vi "Compatibility Pulse Generation.vi"() -> ()   [LabVIEW 2023]
doc: "The Compatibility Pulse Generation example demonstrates how to generate a pulse on an external or RTSI trigger line. Use a pulse to control external events such as triggering a strobe light.\n\nThis example uses the IMAQdx driver to interface with a Camera Link frame grabber. It uses the NI-IMAQdx Compatibility for NI-IMAQ API to facilitate migration between the two drivers. The NI-IMAQdx VIs are drop-in replacements to existing NI-IMAQ VIs."
uses:
  <vilib>/vision/driver/NI_Vision_Acquisition_Software.lvlib
panel:
  in  "Camera Name":refnum<k21> caption="IMAQdx Session"
  in  "Trigger Type":u32(ring) items=["External"=0, "RTSI"=1, "ISO Out"=3]
  in  "Pulse Parameters":T1={"Pulse Delay"=0.1, "Pulse Width"=0.2, "Pulse Polarity"=enum."High True ", "Units"=enum."Seconds"} {"Pulse Width" format="%_6f"; "Pulse Delay" format="%_6f"}
  in  "Signal Type":u32(ring)=4 items=["External"=0, "RTSI "=1, "ISO In"=2, "Status"=4]
  in  "Signal Number":u32
  in  "Status Signal":u32(ring)=16 items=["Acquisition in progress"=15, "Acquisition done"=8, "Horizontal Synchronization Signal"=18, "Vertical Synchronization Signal"=19, "Frame start"=9, "Frame done"=10, "Immediate"=16]
  in  "Trigger Number":u32
  in  "Stop":bool
  out "Image":T2(plugin-control)
  # "Overview: Demonstrates how to generate a pulse or pulse train on one of the external or RTSI trigger lines of a Camera Link frame grabber board.\nRequirements: Vision Acquisition Software 18.0 or later, PCIe-1427, PCIe-1433, PXIe-1435, or PCIe-1437 frame grabber.\nInstructions: \n1. Select the Camera Name.\n2. Run the VI."
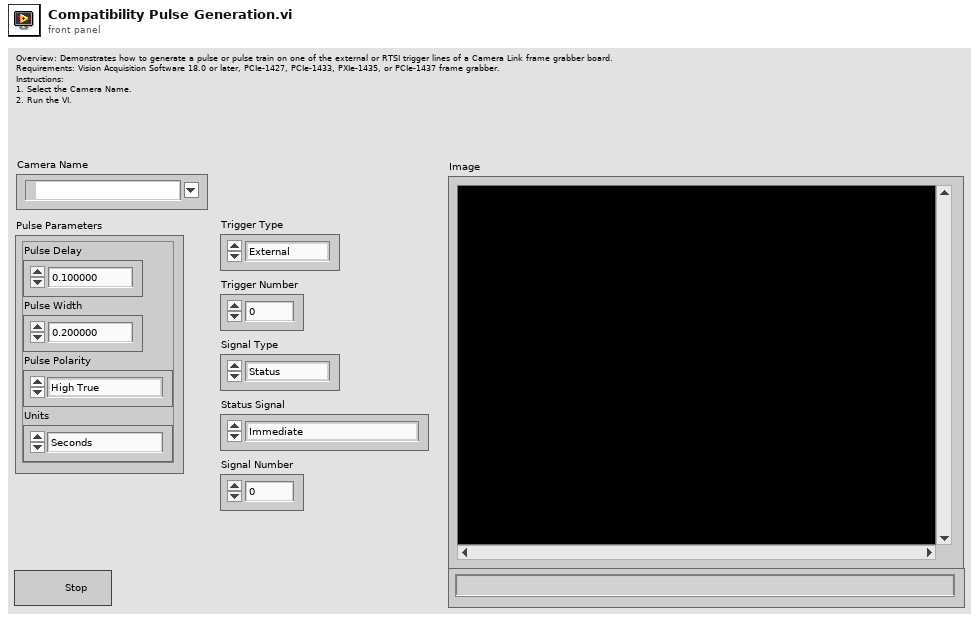
[diagram p1: front panel]
types:
  T1 = cluster{"Pulse Delay":dbl, "Pulse Width":dbl, "Pulse Polarity":enum16{"High True ", "Low True"}, "Units":enum16{"Seconds", "Scaled Encoder Counts"}}
  T2 = typedef "IMAQ Image.ctl" = refnum<image>
  T3 = typedef "IMAQdx.ctl" = refnum<k21>
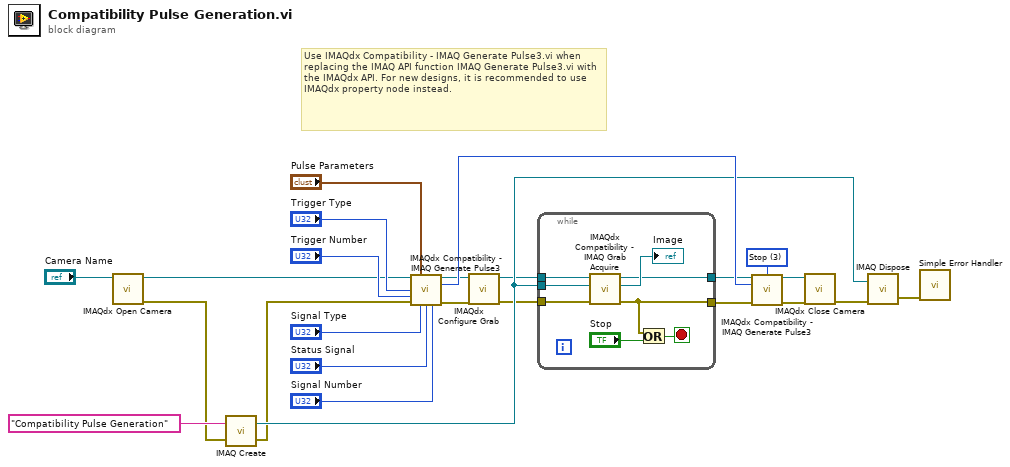
[diagram p0: block diagram]
diagram:
  w23 = u32 3 items=["Pulse train", "Single pulse", "Rearmed pulse", "Stop", "Update"] ("Pulse Mode")
  # "Use IMAQdx Compatibility - IMAQ Generate Pulse3.vi when replacing the IMAQ API function IMAQ Generate Pulse3.vi with the IMAQdx API. For new designs, it is recommended to use IMAQdx property node instead."
  n1 = call <vilib>:"IMAQdx Open Camera.vi"("Session In"="Camera Name") -> ("error out"=w5:errorcluster, "Session Out"=w6:T3)  [unwired: 9 in]
  n2 = call "IMAQ Create"("Image Name"="Compatibility Pulse Generation", "error in (no error)"=w5) -> ("New Image"=w13:T2, "error out"=w8:errorcluster)  [unwired: 2 in, 1 out]
  n3 = call <vilib>:"IMAQdx Compatibility - IMAQ Generate Pulse3.vi"("Session In"=w6, "Pulse Parameters"="Pulse Parameters", "Trigger Type"="Trigger Type", "Trigger Number"="Trigger Number", "error in (no error)"=w8, "Signal Type"="Signal Type", "Status Signal"="Status Signal", "Signal Number"="Signal Number") -> ("Session Out"=w4:T3, "Pulse ID Out"=w20:u32, "error out"=w11:errorcluster)  [unwired: 5 in]
  n4 = call <vilib>:"IMAQdx Configure Grab.vi"("error in"=w11, "Session In"=w4) -> ("error out"=w10:errorcluster, "Session Out"=w9:T3)  [unwired: 8 in]
  n5 = while {
    tunnel: w13 -> [w29]
    tunnel: w10 -> [w30]
    tunnel: w9 -> [w25]
    tunnel: [w27] -> w2
    tunnel: [w26] -> w22
    stop <- w32 stop-if-true
    n6 = call <vilib>:"IMAQdx Compatibility - IMAQ Grab Acquire.vi"("error in (no error)"=w30, "Image In"=w29, "Session In"=w25) -> ("error out"=w26:errorcluster, "Image Out"=→"Image":T2, "Session Out"=w27:T3)  [unwired: 5 in, 1 out]
    n7 = Or(x=w26, y="Stop") -> (x .or. y?=w32:bool)
  }
  n8 = call <vilib>:"IMAQdx Compatibility - IMAQ Generate Pulse3.vi"("Session In"=w2, "Pulse Mode"=w23, "Pulse ID In"=w20, "error in (no error)"=w22) -> ("Session Out"=w3:T3, "error out"=w21:errorcluster)  [unwired: 9 in, 1 out]
  n9 = call <vilib>:"IMAQdx Close Camera.vi"("error in"=w21, "Session In"=w3) -> ("error out"=w24:errorcluster)  [unwired: 9 in]
  n10 = call "IMAQ Dispose"("Image"=w13, "error in (no error)"=w24) -> ("error out"=w7:errorcluster)  [unwired: 1 in, 3 out]
  n11 = call <vilib>:"Simple Error Handler.vi"("error in (no error)"=w7) -> ()  [unwired: 1 in, 8 out]
